vi "WPI_UtilitiesNDE_lv_browse_and_resolve.vi"(0 "serviceTypeName":string="_ni._tcp", 5 "domainName":string, 7 "Browse Timeout (sec)":i32, 9 "Resolve Timeout (sec)":i32=1, 11 "error in":errorcluster, 12 "ifIndices":u32[](array[numeric]), 13 "svcKeyFilters":T1[](array[typedef])) -> (4 "instances":T2[](array[typedef]), 15 "error out":errorcluster)   [LabVIEW 2025]
uses:
  <vilib>/Rock Robotics/WPI/Utilities/mDNSResolveInstance.ctl
  <vilib>/Rock Robotics/WPI/Utilities/ServiceKeyValuePair.ctl
  <vilib>/Rock Robotics/WPI/Utilities/myrio_discovery.dll
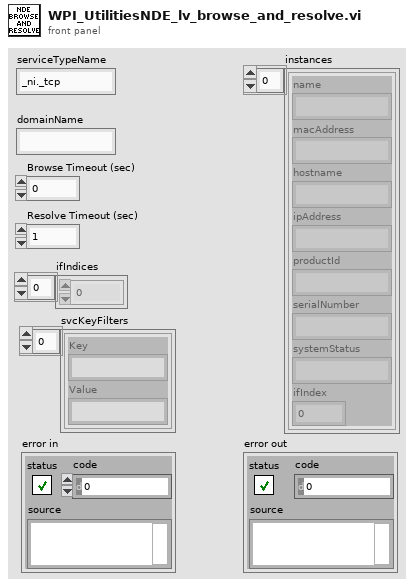
[diagram p1: front panel]
types:
  T1 = typedef "ServiceKeyValuePair.ctl" = cluster{"Key":string, "Value":string}
  T2 = typedef "mdnsResolveInstance.ctl" = cluster{"name":string, "macAddress":string, "hostname":string, "ipAddress":string, "productId":string, "serialNumber":string, "systemStatus":string, "ifIndex":u32}
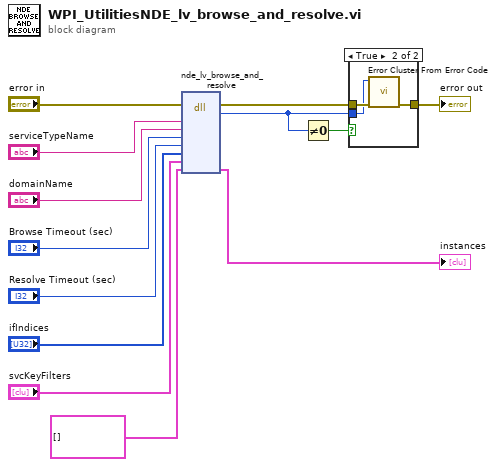
[diagram p0: block diagram]
diagram:
  n1 = dll-call lib="c:/dev/_r/33/src/lvaddon/frc/frcd/FRC_WPILib/objects/labview/win/vi.lib/Rock Robotics/WPI/Utilities/myrio_discovery.dll" fn="nde_lv_browse_and_resolve"(error in="error in", "serviceTypeName"="serviceTypeName", "domainName"="domainName", "browseTimeSec"="Browse Timeout (sec)", "resolveTimeSec"="Resolve Timeout (sec)", "ifIndices"="ifIndices", "svcKeyFilters"="svcKeyFilters", "instances"=T2[] []) -> (error out=w4:errorcluster, "return type"=w2:i32, "instances"=→"instances":T2[])  [unwired: 8 in, 1 out]
  n2 = Not Equal To 0?(x=w2) -> (x != 0?=w3:bool)
  n3 = case shown="True" w3 {
    tunnel: [w14 w17] -> w5
    tunnel: w4 -> [w14 w16]
    tunnel: w2 -> [_ w15]
    frame False {
    }
    frame True {
      n4 = call <vilib>:"Error Cluster From Error Code.vi"("error in (no error)"=w16, "error code (0)"=w15) -> ("error out"=w17:errorcluster)  [unwired: 7 in]
    }
  }
  "error out" <- w5
